vi "SweepType.vi"(0 "VISA IN":refnum<visa-resource-name>, 1 "Sweep Type":string(combo)="LINear", 2 "Start Frq.":dbl=10000000.0, 3 "Stop Frq.":dbl=10000000.0, 4 "Points":dbl=1.0, 5 "error in":errorcluster, 6 "Start Power":i32, 7 "Channel":i32=1, 8 "Stop Power":i32, 9 "CW Frq.":dbl=10000000.0, 10 "CW Frq.":dbl=10000000.0, 11 "Sweep Time(sec)":i32, 13 "Points":dbl=1.0) -> (14 "VISA Out":refnum<visa-resource-name>, 19 "error out":errorcluster)   [LabVIEW 2018, in "PNA-X.lvlib"]
uses:
  PNA-X.lvlib
panel:
  in  "Independent Power Levels? ON/OFF":bool
  in  "Independent IF BW? ON/OFF":bool
  in  "Independent Sweep Time? ON/OFF":bool
  in  "X-Axis Pt. Spacing? ON/OFF":bool
  in  "Allow ARB Segments? ON/OFF":bool
  in  "Show Table?":bool
  in  "Window":i32=1
  # "Segment Sweep Properties"
  # "CW Time Properties"
  # "Power Sweep Properties"
  # "Linear and Log Properties"
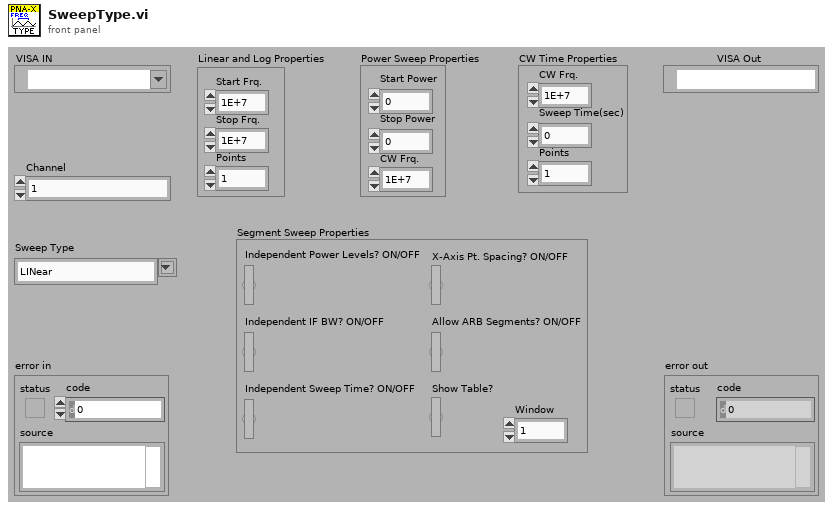
[diagram p1: front panel]
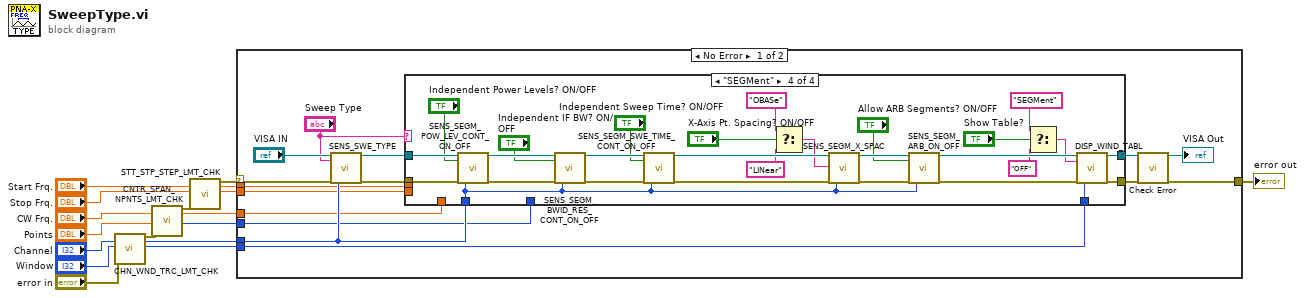
[diagram p0: block diagram]
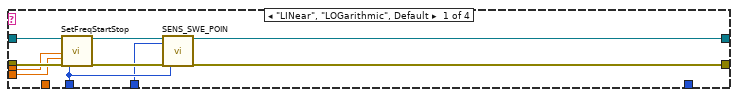
[diagram p2: hidden frame]
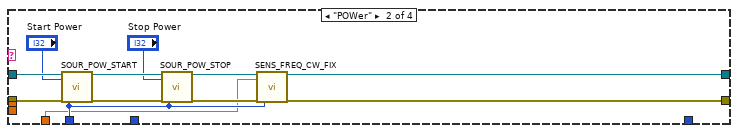
[diagram p3: hidden frame]
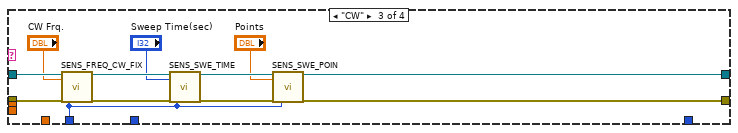
[diagram p4: hidden frame]
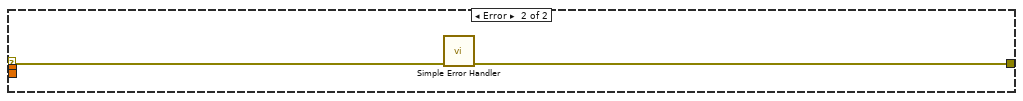
[diagram p5: hidden frame]
diagram:
  n1 = call "CHN_WND_TRC_LMT_CHK.vi"("Channel"="Channel", "Window"="Window", "error in"="error in") -> ("error out"=w17:errorcluster, "Channel"=w8:i32, "Window"=w1:i32)  [unwired: 12 in, 2 out]
  n2 = call "CNTR_SPAN_NPNTS_LMT_CHK.vi"("Center"="CW Frq.", "Npoints"="Points", "error in"=w17) -> ("error out"=w16:errorcluster, "Center"=w4:dbl, "Npoints"=w5:i32)  [unwired: 13 in, 1 out]
  n3 = call "STT_STP_STEP_LMT_CHK.vi"("Start"="Start Frq.", "Stop"="Stop Frq.", "error in"=w16) -> ("error out"=w9:errorcluster, "Start"=w7:dbl, "Stop"=w6:dbl)  [unwired: 13 in, 1 out]
  n4 = case shown="No Error" w9 {
    selector: w9 -> [w30 w96]
    tunnel: [w32 w95] -> w10
    tunnel: w8 -> [w29 _]
    tunnel: w7 -> [w25 _]
    tunnel: w6 -> [w24 _]
    tunnel: w5 -> [w22 _]
    tunnel: w4 -> [w21 _]
    tunnel: w1 -> [w18 _]
    frame No Error {
      n5 = call "SENS_SWE_TYPE.vi"("VISA IN"="VISA IN", "Sweep Type"="Sweep Type", "error in"=w30, "Channel"=w29) -> ("VISA Out"=w27:refnum<visa-resource-name>, "error out"=w26:errorcluster)  [unwired: 14 in]
      n6 = case shown="\"SEGMent\"" "Sweep Type" {
        tunnel: w29 -> [w34 w44 w58 w69]
        tunnel: w27 -> [w42 w51 w62 w87]
        tunnel: w26 -> [w41 w54 w66 w94]
        tunnel: w25 -> [w40 _ _ _]
        tunnel: w24 -> [w39 _ _ _]
        tunnel: [w37 w46 w63 w88] -> w19
        tunnel: [w35 w47 w59 w81] -> w20
        tunnel: w22 -> [w33 _ _ _]
        tunnel: w21 -> [_ w43 _ _]
        tunnel: w18 -> [_ _ _ w80]
        frame "LINear", "LOGarithmic", Default {
          n7 = call "SetFreqStartStop.vi"("VISA IN"=w42, "Start Frequency"=w40, "Stop Frequency"=w39, "error in"=w41, "Channel"=w34) -> ("VISA Out"=w36:refnum<visa-resource-name>, "error out"=w38:errorcluster)  [unwired: 13 in]
          n8 = call "SENS_SWE_POIN.vi"("VISA IN"=w36, "Sweep Points"=w33, "error in"=w38, "Channel"=w34) -> ("VISA Out"=w35:refnum<visa-resource-name>, "error out"=w37:errorcluster)  [unwired: 14 in]
        }
        frame "POWer" {
          n9 = call "SOUR_POW_START.vi"("VISA IN"=w51, "Start Power"="Start Power", "error in"=w54, "Channel"=w44) -> ("VISA Out"=w52:refnum<visa-resource-name>, "error out"=w53:errorcluster)  [unwired: 14 in]
          n10 = call "SOUR_POW_STOP.vi"("VISA IN"=w52, "Stop Power"="Stop Power", "error in"=w53, "Channel"=w44) -> ("VISA Out"=w48:refnum<visa-resource-name>, "error out"=w45:errorcluster)  [unwired: 14 in]
          n11 = call "SENS_FREQ_CW_FIX.vi"("VISA IN"=w48, "CW Frq."=w43, "error in"=w45, "Channel"=w44) -> ("VISA Out"=w47:refnum<visa-resource-name>, "error out"=w46:errorcluster)  [unwired: 14 in]
        }
        frame "CW" {
          n12 = call "SENS_FREQ_CW_FIX.vi"("VISA IN"=w62, "CW Frq."="CW Frq.", "error in"=w66, "Channel"=w58) -> ("VISA Out"=w61:refnum<visa-resource-name>, "error out"=w65:errorcluster)  [unwired: 14 in]
          n13 = call "SENS_SWE_TIME.vi"("VISA IN"=w61, "Sweep Time(sec)"="Sweep Time(sec)", "error in"=w65, "Channel"=w58) -> ("VISA Out"=w60:refnum<visa-resource-name>, "error out"=w64:errorcluster)  [unwired: 14 in]
          n14 = call "SENS_SWE_POIN.vi"("VISA IN"=w60, "Sweep Points"="Points", "error in"=w64, "Channel"=w58) -> ("VISA Out"=w59:refnum<visa-resource-name>, "error out"=w63:errorcluster)  [unwired: 14 in]
        }
        frame "SEGMent" {
          n15 = call "SENS_SEGM_POW_LEV_CONT_ON_OFF.vi"("VISA IN"=w87, "Power Level ON/OFF"="Independent Power Levels? ON/OFF", "error in"=w94, "Channel"=w69) -> ("VISA Out"=w86:refnum<visa-resource-name>, "error out"=w93:errorcluster)  [unwired: 14 in]
          n16 = call "SENS_SEGM_BWID_RES_CONT_ON_OFF.vi"("VISA IN"=w86, "BW Control ON/OFF"="Independent IF BW? ON/OFF", "error in"=w93, "Channel"=w69) -> ("VISA Out"=w85:refnum<visa-resource-name>, "error out"=w92:errorcluster)  [unwired: 14 in]
          n17 = call "SENS_SEGM_SWE_TIME_CONT_ON_OFF.vi"("VISA IN"=w85, "Sweep Time Control ON/OFF"="Independent Sweep Time? ON/OFF", "error in"=w92, "Channel"=w69) -> ("VISA Out"=w84:refnum<visa-resource-name>, "error out"=w91:errorcluster)  [unwired: 14 in]
          n18 = Select(t="OBASe" ("X-Axis Point Spacing(LINear or OBASe)"), s="X-Axis Pt. Spacing? ON/OFF", f="LINear" ("X-Axis Point Spacing(LINear or OBASe)")) -> (s? t:f=w74:string)
          n19 = call "SENS_SEGM_X_SPAC.vi"("VISA IN"=w84, "X-Axis Point Spacing(LINear or OBASe)"=w74, "error in"=w91, "Channel"=w69) -> ("VISA Out"=w83:refnum<visa-resource-name>, "error out"=w90:errorcluster)  [unwired: 14 in]
          n20 = call "SENS_SEGM_ARB_ON_OFF.vi"("VISA IN"=w83, "ARB ON/OFF"="Allow ARB Segments? ON/OFF", "error in"=w90, "Channel"=w69) -> ("VISA Out"=w82:refnum<visa-resource-name>, "error out"=w89:errorcluster)  [unwired: 14 in]
          n21 = Select(t="SEGMent" ("Tables"), s="Show Table?", f="OFF" ("Tables")) -> (s? t:f=w77:string)
          n22 = call "DISP_WIND_TABL.vi"("VISA IN"=w82, "Tables"=w77, "error in"=w89, "Window"=w80) -> ("VISA Out"=w81:refnum<visa-resource-name>, "error out"=w88:errorcluster)  [unwired: 14 in]
        }
      }
      n23 = call "Check Error.vi"("VISA Resource Name"=w20, "error in (no error)"=w19) -> ("dup VISA session"=→"VISA Out":refnum<visa-resource-name>, "error out"=w32:errorcluster)  [unwired: 16 in]
    }
    frame Error {
      n24 = call <vilib>:"Simple Error Handler.vi"("error in (no error)"=w96) -> ("error out"=w95:errorcluster)  [unwired: 4 in, 4 out]
    }
  }
  "error out" <- w10
